vi "LINC Set Packet Configuration.vi"(6 "item formats":T1[](array[typedef]), 7 "item names":string[](array[string]), 8 "error in (no error)":errorcluster, 9 "packet name":string, 10 "type":enum16{"CMD", "TLM"}(ring), 11 "LINC session":refnum<class "LINC.lvclass">) -> (0 "error out":errorcluster, 3 "dup LINC session":refnum<class "LINC.lvclass">)   [LabVIEW 2018, in "STEPkgDriver_LINC.lvlib" / "LINC.lvclass"]
uses:
  LINC.lvclass
  LINC Global Mode.ctl
  STEPkgDriver_LINC.lvlib
  LINC Format Prototype.ctl
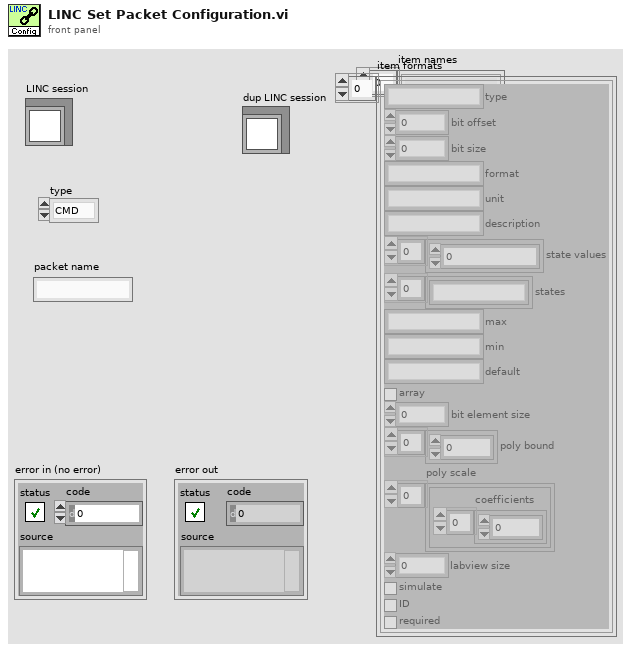
[diagram p1: front panel]
types:
  T1 = typedef "STEPkgDriver_LINC.lvlib/LINC Format Prototype.ctl" = cluster{"type":string, "bit offset":i32, "bit size":i32, "format":string, "unit":string, "description":string, "state values":i64[], "states":string[], "max":string, "min":string, "default":string, "array":bool, "bit element size":i32, "poly bound":dbl[], "poly scale":cluster{"coefficients":dbl[]}[], "labview size":i32, "simulate":bool, "ID":bool, "required":bool}
  T2 = typedef "STEPkgDriver_LINC.lvlib/LINC Global Mode.ctl" = enum16{"INIT", "CLEAR", "ADD_PKT_HDR", "ADD_PKT", "GET_PKT_NAMES", "GET_PKT_DESC", "GET_PKT_HDR", "GET_PKT", "SET_PKT", "SET_DATA", "SIM_EN", "SIM_DS"}
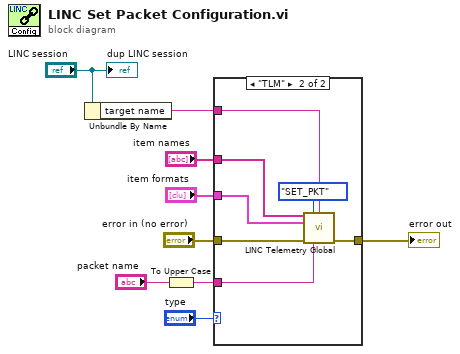
[diagram p0: block diagram]
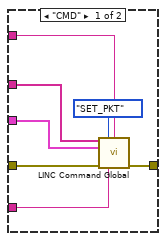
[diagram p2: hidden frame]
diagram:
  n1 = Unbundle By Name("LINC session") -> ("target name"=w7:string)
  n2 = To Upper Case(1:"packet name") -> (0:w3:string)
  n3 = case shown="\"TLM\"" "type" {
    tunnel: "error in (no error)" -> [w15 w22]
    tunnel: [w14 w21] -> w8
    tunnel: w7 -> [w13 w20]
    tunnel: w3 -> [w12 w19]
    tunnel: "item names" -> [w11 w18]
    tunnel: "item formats" -> [w10 w17]
    frame "CMD" {
      n4 = call "LINC Command Global.vi"("item names in"=w11, "mode"=LINC_Global_Mode."SET_PKT", "target name"=w13, "item formats in"=w10, "error in (no error)"=w15, "packet name"=w12) -> ("error out"=w14:errorcluster)  [unwired: 5 in, 4 out]
    }
    frame "TLM" {
      n5 = call "LINC Telemetry Global.vi"("item names in"=w18, "mode"=LINC_Global_Mode."SET_PKT", "target name"=w20, "item formats in"=w17, "error in (no error)"=w22, "packet name"=w19) -> ("error out"=w21:errorcluster)  [unwired: 5 in, 4 out]
    }
  }
  "error out" <- w8
  "dup LINC session" <- "LINC session"
